vi "Initialise Column Headers.vi"(11 "Main Display in":refnum<class "Main Display.lvclass">) -> (0 "error out":errorcluster)   [LabVIEW 2016, in "Assert API Components.lvlib" / "Assert Display.lvlib" / "Main Display.lvlib" / "Main Display.lvclass"]
uses:
  Main Display.lvclass
  C:/Program Files (x86)/National Instruments/LabVIEW 2016/vi.lib/ActorFramework/Actor/Actor.lvclass
  Actions.ctl
  <vilib>/ActorFramework/Actor/Actor.lvclass/Actor.ctl
  <vilib>/ActorFramework/Message Enqueuer/Message Enqueuer.lvclass/Message Enqueuer.ctl
  Main Display.lvclass/Main Display.ctl
  Display Configurations/Base Display Configuration.lvclass/Base Display Configuration.ctl
  Main Display Messages/Do Action Msg/Do Action Msg.lvclass/Do Action Msg.ctl
  <vilib>/ActorFramework/Message Enqueuer/Init from Existing Queue.vi
  <vilib>/ActorFramework/Message Enqueuer/Enqueue.vi
  Main Display Messages/Do Action Msg/Do Action Msg.lvclass
  C:/Program Files (x86)/National Instruments/LabVIEW 2016/vi.lib/ActorFramework/Message/Message.lvclass
  <vilib>/Utility/LVClass/Get LV Class Name.vi
  <resource>/AFDebug/Generate Trace for Message.vi
  <vilib>/ActorFramework/Message Priority Queue/Priority Enqueue.vi
  <vilib>/ActorFramework/Message Enqueuer/Message Enqueuer.lvclass
  <vilib>/ActorFramework/Actor/Actor.lvclass
  Display Configurations/Base Display Configuration.lvclass
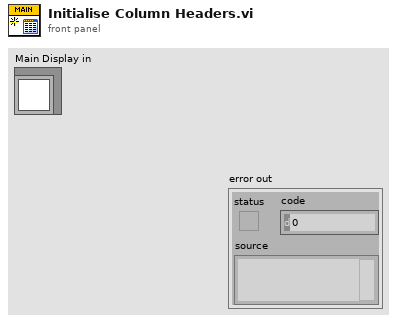
[diagram p1: front panel]
types:
  T1 = typedef "Assert API Components.lvlib/Assert Display.lvlib/Main Display.lvlib/Main Display.lvclass/Actions.ctl" = enum16{"Update Column Headers", "Update Timeout"}
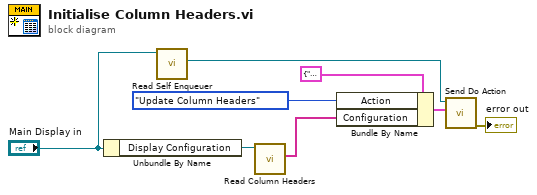
[diagram p0: block diagram]
diagram:
  n1 = Unbundle By Name("Main Display in") -> ("Display Configuration"=w3:refnum<class "Base Display Configuration.lvclass">)
  n2 = call <vilib>:"Read Self Enqueuer.vi"("Actor"="Main Display in") -> ("Self Enqueuer"=w7:refnum<class "Message Enqueuer.lvclass">)  [unwired: 10 in]
  n3 = call "Read Column Headers.vi"("Base Display Configuration in"=w3) -> ("Column Headers"=w2:string[])  [unwired: 10 in]
  n4 = Bundle By Name(cluster=cluster{"Action":T1, "Configuration":variant} {"Action"=enum."Update Column Headers", "Configuration"=variant} ("Action Configuration"), "Action"=Actions."Update Column Headers", "Configuration"=w2) -> (w5:cluster{"Action":T1, "Configuration":variant})
  n5 = call "Send Do Action.vi"("Action Configuration"=w5, "Message Enqueuer"=w7) -> ("error out"=→"error out":errorcluster)  [unwired: 8 in, 1 out]
